vi "E4981_command - 複製.vi"(8 "error in (no error)":errorcluster, 10 "input":T1={"Frequency (1:1kHz)"=1, "Frequency Shift (2: 0%)"=2, "Range"=enum."1p"} {"Frequency Shift (2: 0%)" items=["-2%", "-1%", "0%", "1%", "2%"]; "Frequency (1:1kHz)" items=["120 Hz Frequency", "1 kHz Frequency", "1 MHz Frequency"]}, 11 "command":T3(ring)) -> (0 "error out":errorcluster, 1 "bin":i32, 3 "output":T2={"connectd"=TRUE, "CAP cab"=0.0, "DF  Cab"=0.0} {"CAP cab" format="%#_6p"})   [LabVIEW 2016]
uses:
  meter global.vi
  AOIFramwork/AOIFramework.lvlib
panel:
  in  "reset":bool
  # "CAP DF 電錶作業中"
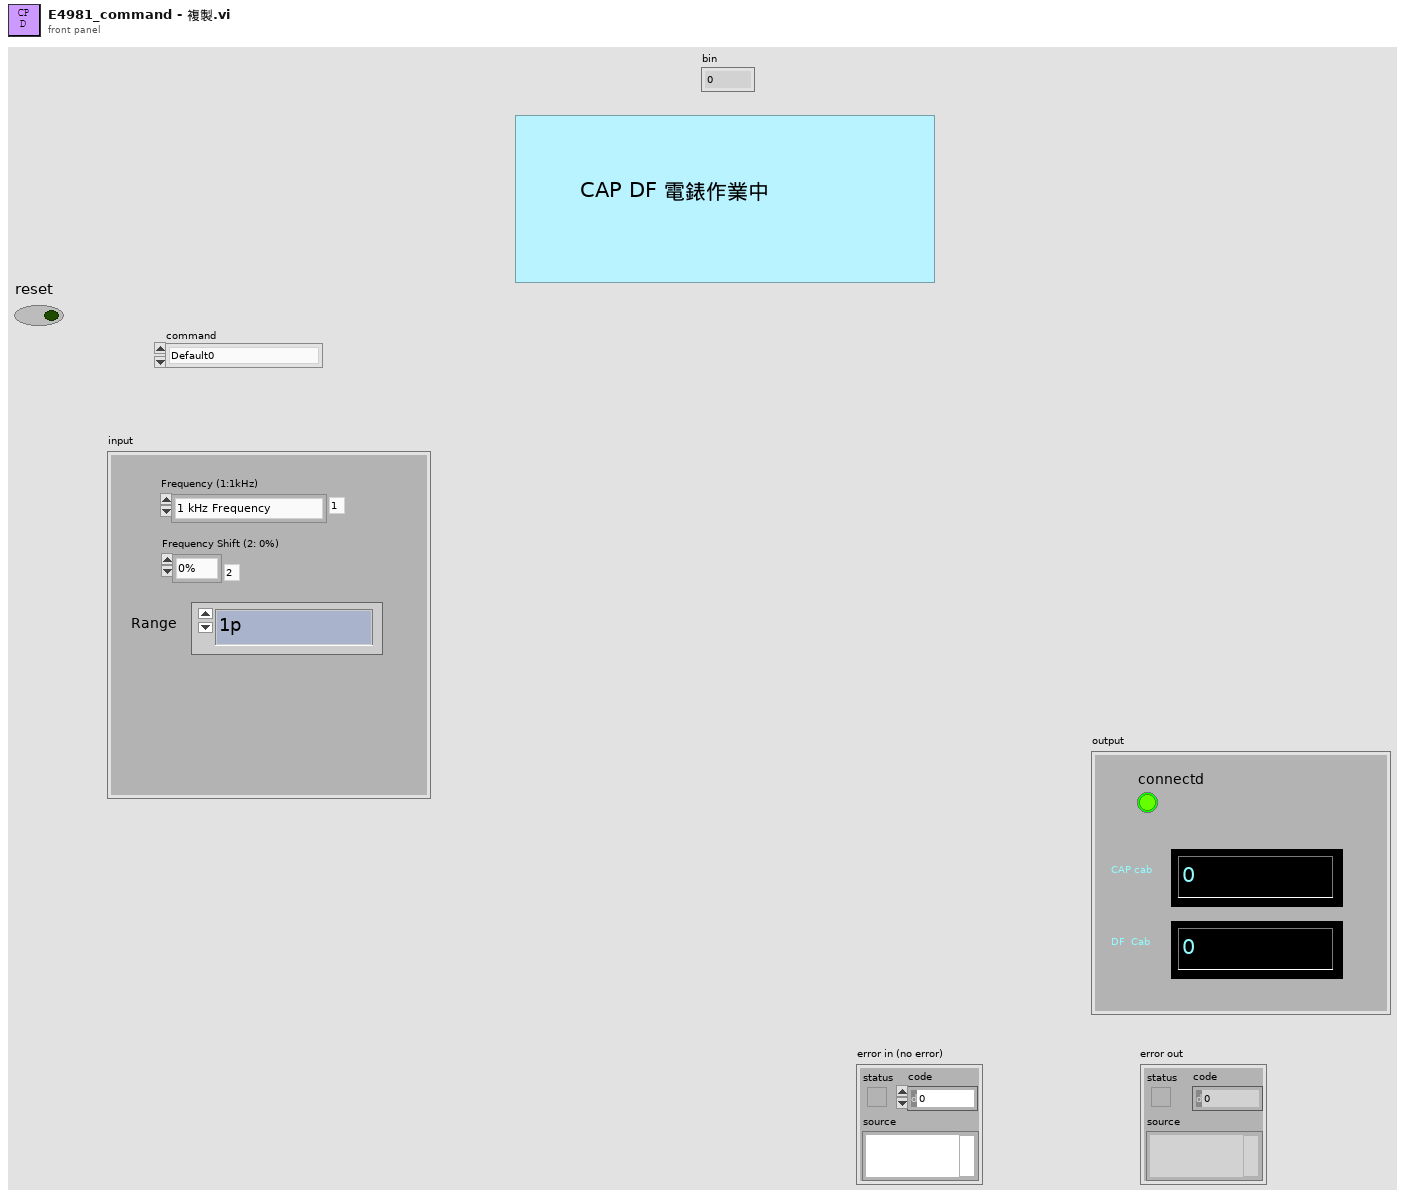
[diagram p1: front panel]
types:
  T1 = cluster{"Frequency (1:1kHz)":u16, "Frequency Shift (2: 0%)":u16, "Range":enum16{"1p", "2.2p", "4.7p", "10p", "22p", "47p", "100p", "220p", "470p", "1n", "2.2n", "4.7n", "10n", "22n", "47n", "100n", "220n", "470n", "1u", "2.2u", "4.7u", "10u", "22u", "47u", "100u", "220u", "470u", "1m", "AUTO", ""}}
  T2 = cluster{"connectd":bool, "CAP cab":dbl, "DF  Cab":dbl}
  T3 = enum16{"Default0", "checkconnect", "int", "changeFEQ", "changeRange", "trigger", "triggerauto"}
  T4 = enum16{"1p", "2.2p", "4.7p", "10p", "22p", "47p", "100p", "220p", "470p", "1n", "2.2n", "4.7n", "10n", "22n", "47n", "100n", "220n", "470n", "1u", "2.2u", "4.7u", "10u", "22u", "47u", "100u", "220u", "470u", "1m", "AUTO", ""}
  T5 = typedef "TypeDef_PNData.ctl" = cluster{"External Diameter":dbl, "Height":dbl, "Range":enum16{"1p", "2.2p", "4.7p", "10p", "22p", "47p", "100p", "220p", "470p", "1n", "2.2n", "4.7n", "10n", "22n", "47n", "100n", "220n", "470n", "1u", "2.2u", "4.7u", "10u", "22u", "47u", "100u", "220u", "470u", "1m", "AUTO", ""}, "DFmin":dbl, "Cap_num":dbl, "F":u16, "BIN3+":dbl, "BIN3- ":dbl, "BIN2+":dbl, "BIN2-":dbl, "BIN1+":dbl, "BIN1-":dbl, "Frequencies":enum16{"120HZ", "1K  HZ", "1M HZ"}, "DFmax":dbl, "Part_5":dbl, "Part_6":dbl, "Part_4":dbl, "Part_8":dbl, "Part_7":dbl, "Par_2":dbl, "part_1":enum16{"DC", "AC"}, "Part_9":dbl, "Part_18":dbl, "Part_15":dbl, "Part_13":dbl, "Part_14":dbl, "Part_16":dbl, "Internal Diameter":dbl}
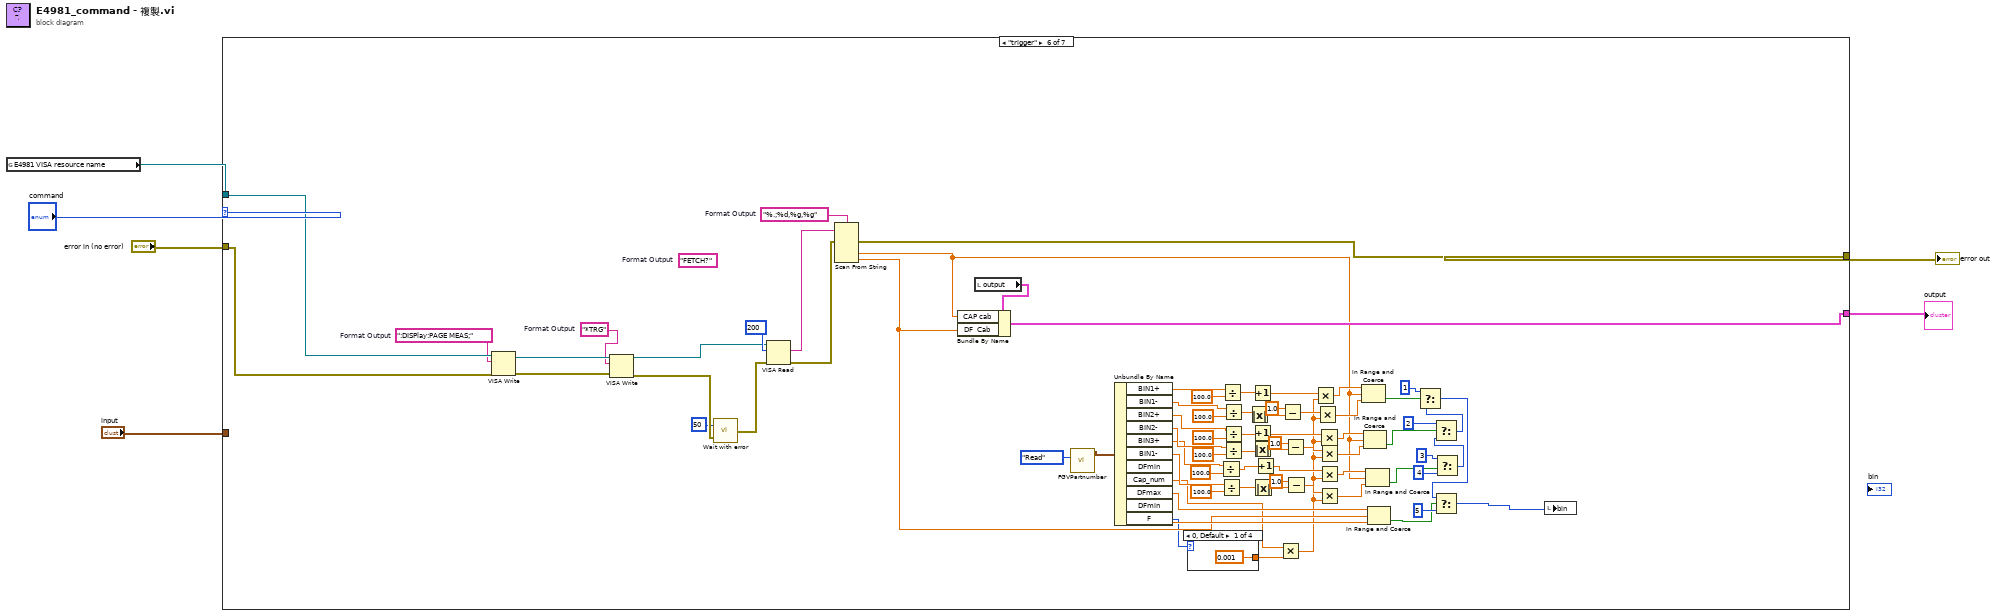
[diagram p0: block diagram]
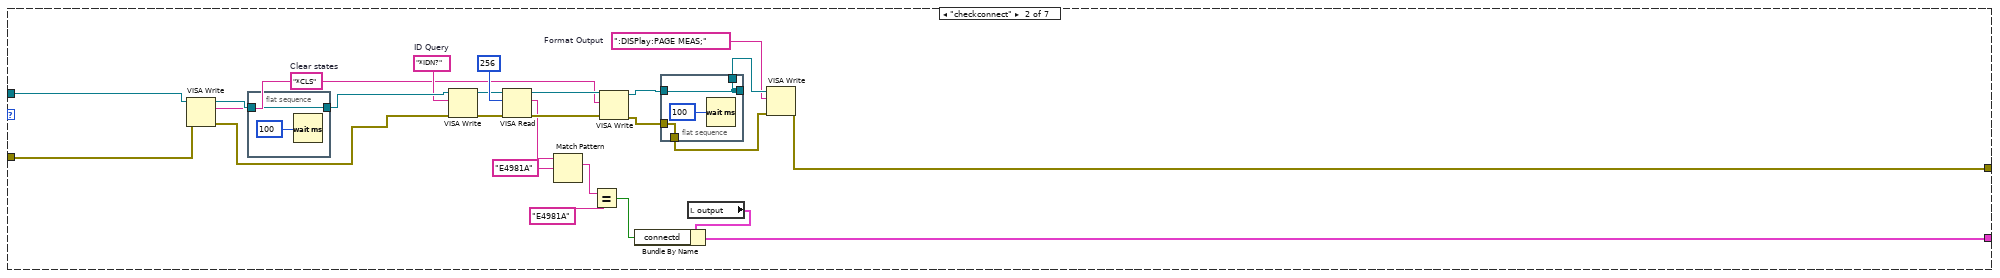
[diagram p3: hidden frame]
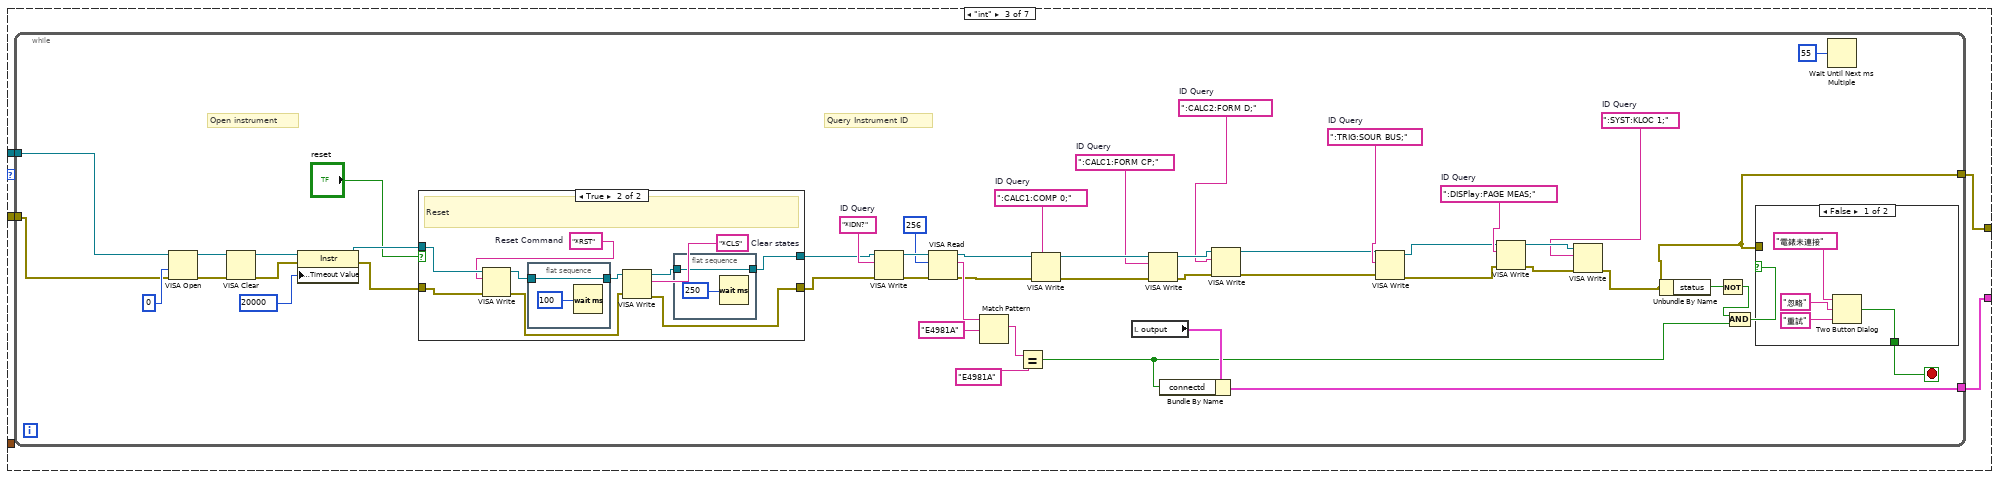
[diagram p4: hidden frame]
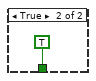
[diagram p6: hidden frame]
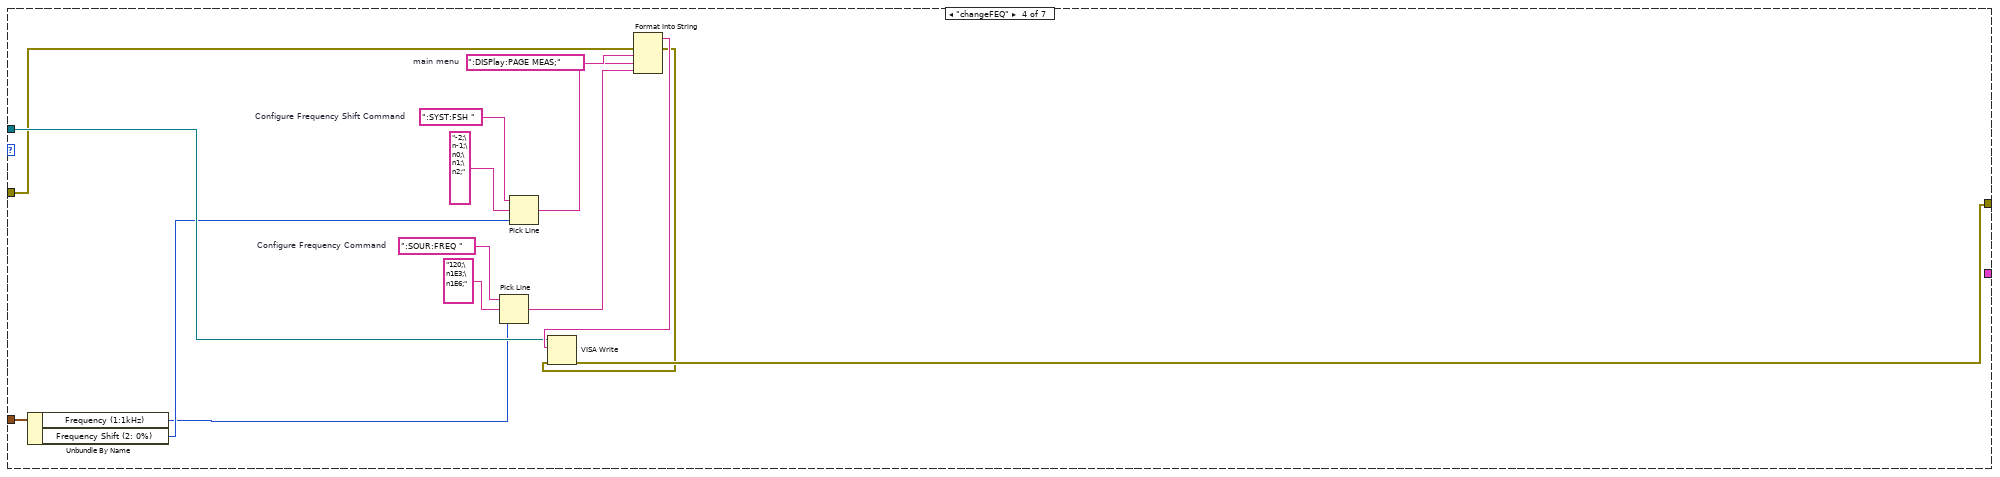
[diagram p7: hidden frame]
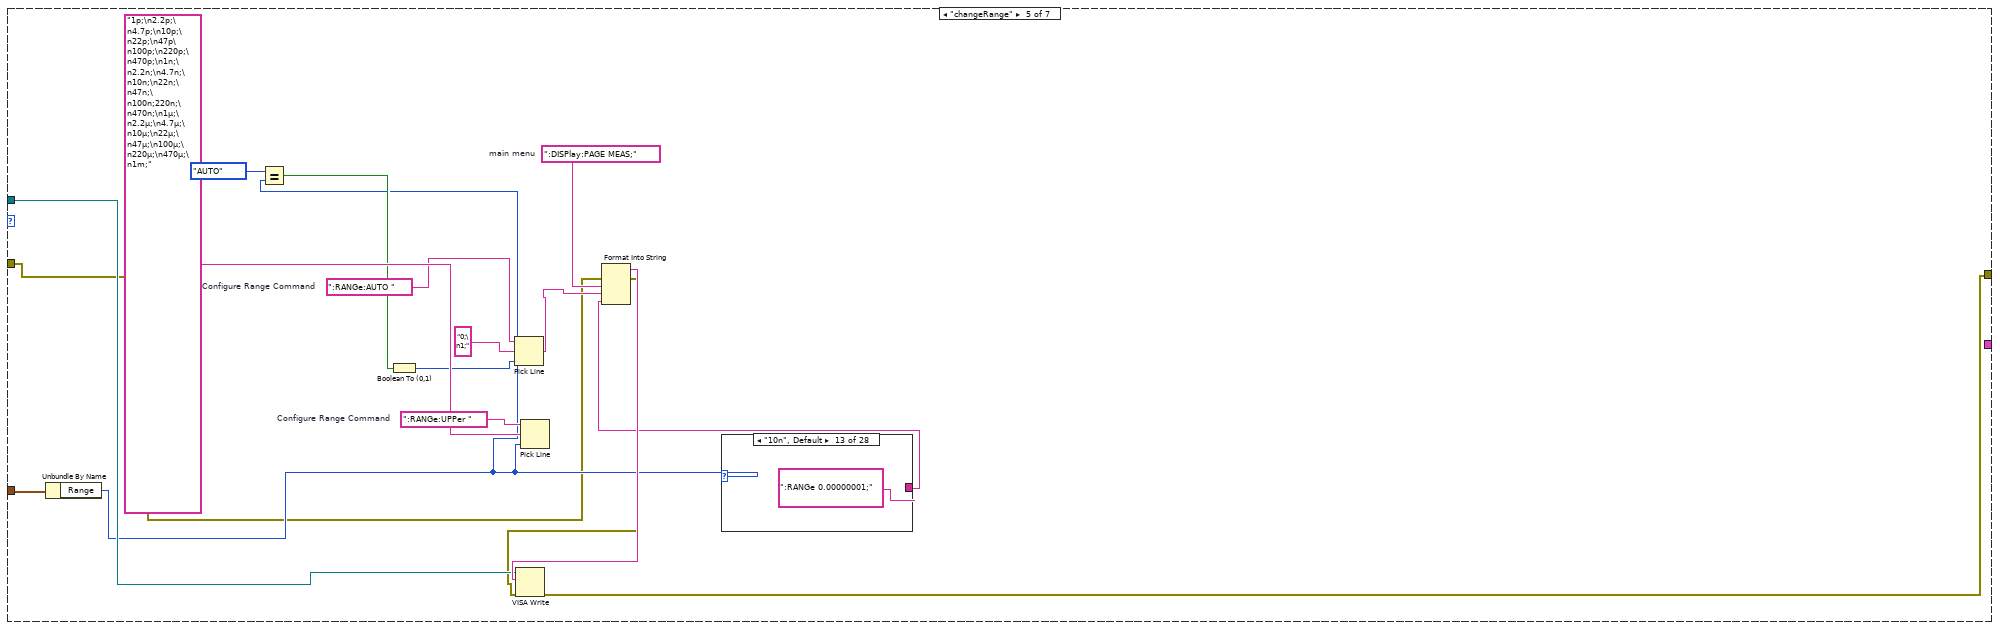
[diagram p8: hidden frame]
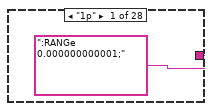
[diagram p9: hidden frame]
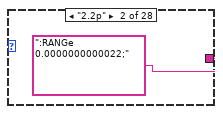
[diagram p10: hidden frame]
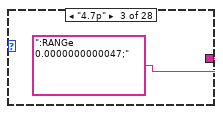
[diagram p11: hidden frame]
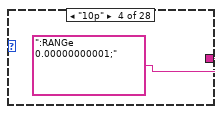
[diagram p12: hidden frame]
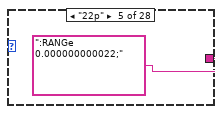
[diagram p13: hidden frame]
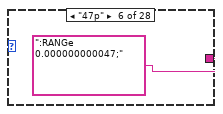
[diagram p14: hidden frame]
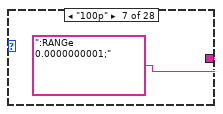
[diagram p15: hidden frame]
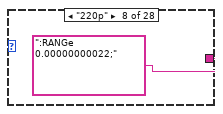
[diagram p16: hidden frame]
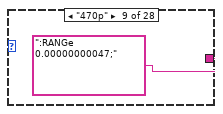
[diagram p17: hidden frame]
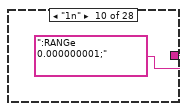
[diagram p18: hidden frame]
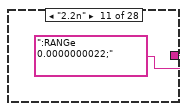
[diagram p19: hidden frame]
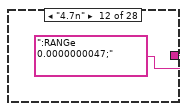
[diagram p20: hidden frame]
diagram:
  n1 = global read "meter global.vi" "E4981 VISA resource name"() -> (w4:refnum<visa-resource-name>)
  n2 = case shown="\"trigger\"" "command" {
    tunnel: "error in (no error)" -> [_ w13 w38 w111 w126 w237 w316]
    tunnel: [_ w12 w40 w115 w129 w232 w258] -> w5
    tunnel: w4 -> [_ w10 w39 w116 w130 w238 w317]
    tunnel: [_ w7 w37 _ _ w235 w314] -> w2
    tunnel: "input" -> [_ _ _ w114 w128 _ _]
    frame "Default0", Default {
    }
    frame "checkconnect" {
      w27 = ":DISPlay:PAGE MEAS;"  # Format Output
      w11 = "*CLS"  # Clear states
      w19 = "*IDN?"  # ID Query
      n3 = VISA Write(VISA resource name=w10, write buffer=w11, error in (no error)=w13) -> (VISA resource name out=w24:refnum<visa-resource-name>, error out=w23:errorcluster)  [unwired: 1 out]
      n4 = flat-sequence {
        tunnel: [w35] -> w22
        tunnel: w24 -> [w35]
        frame #0 {
          n5 = Wait (ms)(milliseconds to wait=u32 100) -> ()  [unwired: 1 out]
        }
      }
      n6 = VISA Write(VISA resource name=w22, write buffer=w19, error in (no error)=w23) -> (VISA resource name out=w15:refnum<visa-resource-name>, error out=w16:errorcluster)  [unwired: 1 out]
      n7 = VISA Read(VISA resource name=w15, byte count=u32 256, error in (no error)=w16) -> (VISA resource name out=w25:refnum<visa-resource-name>, read buffer=w14:string, error out=w26:errorcluster)  [unwired: 1 out]
      n8 = Match Pattern(string=w14, regular expression="E4981A") -> (match substring=w20:string)  [unwired: 1 in, 3 out]
      n9 = Equal?(x=w20, y="E4981A") -> (x = y?=w8:bool)
      n10 = VISA Write(VISA resource name=w25, write buffer=w11, error in (no error)=w26) -> (VISA resource name out=w28:refnum<visa-resource-name>, error out=w29:errorcluster)  [unwired: 1 out]
      n11 = flat-sequence {
        tunnel: [w32] -> _
        tunnel: w28 -> [w32]
        tunnel: w29 -> [w33]
        tunnel: [w33] -> w30
        tunnel: [w32] -> w31
        frame #0 {
          n12 = Wait (ms)(milliseconds to wait=u32 100) -> ()  [unwired: 1 out]
        }
      }
      n13 = local read "output"() -> (w9:T2)
      n14 = Bundle By Name(cluster=w9, "connectd"=w8) -> (w7:T2)
      n15 = VISA Write(VISA resource name=w31, write buffer=w27, error in (no error)=w30) -> (error out=w12:errorcluster)  [unwired: 2 out]
    }
    frame "int" {
      n16 = while {
        tunnel: [w46] -> w40
        tunnel: w39 -> [w45]
        tunnel: w38 -> [w44]
        tunnel: [w41] -> w37
        stop <- w73 stop-if-true
        w54 = ":TRIG:SOUR BUS;"  # ID Query
        w57 = ":SYST:KLOC 1;"  # ID Query
        w60 = ":DISPlay:PAGE MEAS;"  # ID Query
        w61 = ":CALC2:FORM D;"  # ID Query
        w62 = ":CALC1:FORM CP;"  # ID Query
        w71 = ":CALC1:COMP 0;"  # ID Query
        w77 = "*IDN?"  # ID Query
        # "Query Instrument ID"
        # "Open instrument"
        n17 = VISA Open(access mode=u32 0, error in (no error)=w44, VISA resource name=w45) -> (VISA resource name=w86:refnum<visa-resource-name>, error out=w85:errorcluster)  [unwired: 2 in]
        n18 = VISA Clear(VISA resource name=w86, error in (no error)=w85) -> (VISA resource name out=w84:refnum<visa-resource-name>, error out=w83:errorcluster)
        n19 = property class="Instr"(reference=w84, error in=w83, "General Settings:Timeout Value"=u32 20000) -> (reference out=w50:refnum<visa-resource-name>, error out=w48:errorcluster)
        n20 = case shown="True" "reset" {
          tunnel: [w90 w95] -> w51
          tunnel: w50 -> [w90 w100]
          tunnel: [w89 w93] -> w49
          tunnel: w48 -> [w89 w92]
          frame False {
          }
          frame True {
            w91 = "*CLS"  # Clear states
            w99 = "*RST"  # Reset Command
            # "Reset"
            n21 = VISA Write(VISA resource name=w100, write buffer=w99, error in (no error)=w92) -> (VISA resource name out=w97:refnum<visa-resource-name>, error out=w94:errorcluster)  [unwired: 1 out]
            n22 = flat-sequence {
              tunnel: [w103] -> w98
              tunnel: w97 -> [w103]
              frame #0 {
                n23 = Wait (ms)(milliseconds to wait=u32 100) -> ()  [unwired: 1 out]
              }
            }
            n24 = VISA Write(VISA resource name=w98, write buffer=w91, error in (no error)=w94) -> (VISA resource name out=w96:refnum<visa-resource-name>, error out=w93:errorcluster)  [unwired: 1 out]
            n25 = flat-sequence {
              tunnel: [w101] -> w95
              tunnel: w96 -> [w101]
              frame #0 {
                n26 = Wait (ms)(milliseconds to wait=u32 250) -> ()  [unwired: 1 out]
              }
            }
          }
        }
        n27 = VISA Write(VISA resource name=w51, write buffer=w77, error in (no error)=w49) -> (VISA resource name out=w81:refnum<visa-resource-name>, error out=w80:errorcluster)  [unwired: 1 out]
        n28 = VISA Read(VISA resource name=w81, byte count=u32 256, error in (no error)=w80) -> (VISA resource name out=w69:refnum<visa-resource-name>, read buffer=w82:string, error out=w70:errorcluster)  [unwired: 1 out]
        n29 = Match Pattern(string=w82, regular expression="E4981A") -> (match substring=w75:string)  [unwired: 1 in, 3 out]
        n30 = Equal?(x=w75, y="E4981A") -> (x = y?=w42:bool)
        n31 = VISA Write(VISA resource name=w69, write buffer=w71, error in (no error)=w70) -> (VISA resource name out=w66:refnum<visa-resource-name>, error out=w65:errorcluster)  [unwired: 1 out]
        n32 = local read "output"() -> (w43:T2)
        n33 = VISA Write(VISA resource name=w66, write buffer=w62, error in (no error)=w65) -> (VISA resource name out=w63:refnum<visa-resource-name>, error out=w64:errorcluster)  [unwired: 1 out]
        n34 = Bundle By Name(cluster=w43, "connectd"=w42) -> (w41:T2)
        n35 = VISA Write(VISA resource name=w63, write buffer=w61, error in (no error)=w64) -> (VISA resource name out=w53:refnum<visa-resource-name>, error out=w52:errorcluster)  [unwired: 1 out]
        n36 = VISA Write(VISA resource name=w53, write buffer=w54, error in (no error)=w52) -> (VISA resource name out=w56:refnum<visa-resource-name>, error out=w55:errorcluster)  [unwired: 1 out]
        n37 = VISA Write(VISA resource name=w56, write buffer=w60, error in (no error)=w55) -> (VISA resource name out=w58:refnum<visa-resource-name>, error out=w59:errorcluster)  [unwired: 1 out]
        n38 = VISA Write(VISA resource name=w58, write buffer=w57, error in (no error)=w59) -> (error out=w46:errorcluster)  [unwired: 2 out]
        n39 = Unbundle By Name(w46) -> ("status"=w68:bool)
        n40 = Not(x=w68) -> (.not. x?=w67:bool)
        n41 = And(x=w67, y=w42) -> (x .and. y?=w76:bool)
        n42 = case shown="False" w76 {
          tunnel: [w107 TRUE ("cancel 2")] -> w73
          tunnel: w46 -> [_ _]
          frame False {
            n43 = Two Button Dialog(message="電錶未連接", 1:"重試" ("T button name (\"OK\")"), 2:"忽略" ("F button name (\"Cancel\")")) -> (T button?=w107:bool)
          }
          frame True {
          }
        }
        n44 = Wait Until Next ms Multiple(millisecond multiple=u32 55) -> ()  [unwired: 1 out]
      }
    }
    frame "changeFEQ" {
      w120 = ":DISPlay:PAGE MEAS;"  # main menu
      w121 = ":SYST:FSH "  # Configure Frequency Shift Command
      w122 = ":SOUR:FREQ "  # Configure Frequency Command
      n45 = Unbundle By Name(w114) -> ("Frequency (1:1kHz)"=w112:u16, "Frequency Shift (2: 0%)"=w113:u16)
      n46 = Pick Line(string ("")=w122, multi-line string="120;\n1E3;\n1E6;", line index=w112) -> (output string=w118:string)
      n47 = Pick Line(string ("")=w121, multi-line string="-2;\n-1;\n0;\n1;\n2;", line index=w113) -> (output string=w119:string)
      n48 = Format Into String(error in=w111, w120, w119, w118) -> (resulting string=w117:string, error out=w110:errorcluster)  [unwired: 2 in]
      n49 = VISA Write(VISA resource name=w116, write buffer=w117, error in (no error)=w110) -> (error out=w115:errorcluster)  [unwired: 2 out]
    }
    frame "changeRange" {
      w139 = ":RANGe:UPPer "  # Configure Range Command
      w136 = ":RANGe:AUTO "  # Configure Range Command
      w141 = ":DISPlay:PAGE MEAS;"  # main menu
      n50 = Unbundle By Name(w128) -> ("Range"=w127:T4)
      n51 = Equal?(x=T4."AUTO", y=w127) -> (x = y?=w134:bool)
      n52 = Boolean To (0,1)(Boolean=w134) -> (0, 1=w133:i16)
      n53 = Pick Line(string ("")=w136, multi-line string="0;\n1;", line index=w133) -> (output string=w132:string)
      n54 = Pick Line(string ("")=w139, multi-line string="1p;\n2.2p;\n4.7p;\n10p;\n22p;\n47p\n100p;\n220p;\n470p;\n1n;\n2.2n;\n4.7n;\n10n;\n22n;\n47n;\n100n;220n;\n470n;\n1μ;\n2.2μ;\n4.7μ;\n10μ;\n22μ;\n47μ;\n100μ;\n220μ;\n470μ;\n1m;", line index=w127) -> ()  [unwired: 1 out]
      n55 = case shown="\"10n\", Default" w127 {
        tunnel: [":RANGe 0.000000000001;" ("Configure Range Command") ":RANGe 0.0000000000022;" ("Configure Range Command") ":RANGe 0.0000000000047;" ("Configure Range Command") ":RANGe 0.00000000001;" ("Configure Range Command") ":RANGe 0.000000000022;" ("Configure Range Command") ":RANGe 0.000000000047;" ("Configure Range Command") ":RANGe 0.0000000001;" ("Configure Range Command") ":RANGe 0.00000000022;" ("Configure Range Command") ":RANGe 0.00000000047;" ("Configure Range Command") ":RANGe 0.000000001;" ("Configure Range Command") ":RANGe 0.0000000022;" ("Configure Range Command") ":RANGe 0.0000000047;" ("Configure Range Command") ":RANGe 0.00000001;" ("Configure Range Command") ":RANGe 0.000000022;" ("Configure Range Command") ":RANGe 0.000000047;" ("Configure Range Command") ":RANGe 0.0000001;" ("Configure Range Command") ":RANGe 0.00000022;" ("Configure Range Command") ":RANGe 0.00000047;" ("Configure Range Command") ":RANGe 0.000001;" ("Configure Range Command") ":RANGe 0.0000022;" ("Configure Range Command") ":RANGe 0.0000047;" ("Configure Range Command") ":RANGe 0.00001;" ("Configure Range Command") ":RANGe 0.000022;" ("Configure Range Command") ":RANGe 0.000047;" ("Configure Range Command") ":RANGe 0.0001;" ("Configure Range Command") ":RANGe 0.00022;" ("Configure Range Command") ":RANGe 0.00047;" ("Configure Range Command") ":RANGe 0.001;" ("Configure Range Command")] -> w131
        frame "1p" {
        }
        frame "2.2p" {
        }
        frame "4.7p" {
        }
        frame "10p" {
        }
        frame "22p" {
        }
        frame "47p" {
        }
        frame "100p" {
        }
        frame "220p" {
        }
        frame "470p" {
        }
        frame "1n" {
        }
        frame "2.2n" {
        }
        frame "4.7n" {
        }
        frame "10n", Default {
        }
        frame "22n" {
        }
        frame "47n" {
        }
        frame "100n" {
        }
        frame "220n" {
        }
        frame "470n" {
        }
        frame "1u" {
        }
        frame "2.2u" {
        }
        frame "4.7u" {
        }
        frame "10u" {
        }
        frame "22u" {
        }
        frame "47u" {
        }
        frame "100u" {
        }
        frame "220u" {
        }
        frame "470u" {
        }
        frame "1m" {
        }
      }
      n56 = Format Into String(error in=w126, w141, w132, w131) -> (resulting string=w140:string, error out=w125:errorcluster)  [unwired: 2 in]
      n57 = VISA Write(VISA resource name=w130, write buffer=w140, error in (no error)=w125) -> (error out=w129:errorcluster)  [unwired: 2 out]
    }
    frame "trigger" {
      w234 = ":DISPlay:PAGE MEAS;"  # Format Output
      (unwired) "FETCH?"  # Format Output
      w239 = "*TRG"  # Format Output
      w243 = "%.;%d,%g,%g"  # Format Output
      n58 = VISA Write(VISA resource name=w238, write buffer=w234, error in (no error)=w237) -> (VISA resource name out=w240:refnum<visa-resource-name>, error out=w241:errorcluster)  [unwired: 1 out]
      n59 = VISA Write(VISA resource name=w240, write buffer=w239, error in (no error)=w241) -> (VISA resource name out=w242:refnum<visa-resource-name>, error out=w172:errorcluster)  [unwired: 1 out]
      n60 = call "Wait with error.vi"("error in (no error)"=w172, "milliseconds to wait"=u32 50) -> ("error out"=w171:errorcluster)
      n61 = VISA Read(VISA resource name=w242, byte count=u32 200, error in (no error)=w171) -> (read buffer=w244:string, error out=w233:errorcluster)  [unwired: 2 out]
      n62 = Scan From String(format string=w243, input string=w244, error in=w233) -> (error out=w232:errorcluster, output 2=w178:dbl, output 3=w177:dbl)  [unwired: 5 in, 2 out]
      n63 = local read "output"() -> (w236:T2)
      n64 = Bundle By Name(cluster=w236, "CAP cab"=w178, "DF  Cab"=w177) -> (w235:T2)
      n65 = call "FGVPartnumber.vi"("Enum"=enum16{"Write", "Read"}."Read") -> ("UnitParamiterCluster out"=w230:T5)  [unwired: 10 in]
      n66 = Unbundle By Name(w230) -> ("BIN1+"=w229:dbl, "BIN1-"=w226:dbl, "BIN2+"=w224:dbl, "BIN2-"=w222:dbl, "BIN3+"=w220:dbl, "BIN1-"=w218:dbl, "Cap_num"=w174:dbl, "DFmax"=w193:dbl, "DFmin"=w192:dbl, "F"=w176:u16)  [unwired: 1 out]
      n67 = case shown="0, Default" w176 {
        tunnel: [0.001 1e-06 1e-09 1e-12] -> w175
        frame 0, Default {
        }
        frame 1 {
        }
        frame 2 {
        }
        frame 3 {
        }
      }
      n68 = Divide(x=w220, y=100.0) -> (x/y=w206:dbl)
      n69 = Divide(x=w218, y=100.0) -> (x/y=w208:dbl)
      n70 = Divide(x=w229, y=100.0) -> (x/y=w217:dbl)
      n71 = Divide(x=w226, y=100.0) -> (x/y=w216:dbl)
      n72 = Divide(x=w224, y=100.0) -> (x/y=w207:dbl)
      n73 = Divide(x=w222, y=100.0) -> (x/y=w211:dbl)
      n74 = Absolute Value(x=w216) -> (abs(x)=w215:dbl)
      n75 = Increment(x=w217) -> (x+1=w205:dbl)
      n76 = Increment(x=w207) -> (x+1=w203:dbl)
      n77 = Absolute Value(x=w211) -> (abs(x)=w212:dbl)
      n78 = Absolute Value(x=w208) -> (abs(x)=w210:dbl)
      n79 = Increment(x=w206) -> (x+1=w201:dbl)
      n80 = Multiply(x=w174, y=w175) -> (x*y=w173:dbl)
      n81 = Subtract(x=1.0, y=w215) -> (x-y=w204:dbl)
      n82 = Subtract(x=1.0, y=w212) -> (x-y=w202:dbl)
      n83 = Subtract(x=1.0, y=w210) -> (x-y=w200:dbl)
      n84 = Multiply(x=w205, y=w173) -> (x*y=w199:dbl)
      n85 = Multiply(x=w204, y=w173) -> (x*y=w198:dbl)
      n86 = Multiply(x=w203, y=w173) -> (x*y=w197:dbl)
      n87 = Multiply(x=w202, y=w173) -> (x*y=w196:dbl)
      n88 = Multiply(x=w201, y=w173) -> (x*y=w195:dbl)
      n89 = Multiply(x=w200, y=w173) -> (x*y=w194:dbl)
      n90 = In Range and Coerce(upper limit=w199, x=w178, lower limit=w198) -> (In Range?=w191:bool)  [unwired: 1 out]
      n91 = In Range and Coerce(upper limit=w197, x=w178, lower limit=w196) -> (In Range?=w183:bool)  [unwired: 1 out]
      n92 = In Range and Coerce(upper limit=w195, x=w178, lower limit=w194) -> (In Range?=w185:bool)  [unwired: 1 out]
      n93 = In Range and Coerce(upper limit=w193, x=w177, lower limit=w192) -> (In Range?=w186:bool)  [unwired: 1 out]
      n94 = Select(t=3, s=w185, f=4) -> (s? t:f=w184:i32)
      n95 = Select(t=2, s=w183, f=w184) -> (s? t:f=w182:i32)
      n96 = Select(t=1, s=w191, f=w182) -> (s? t:f=w180:i32)
      n97 = Select(t=w180, s=w186, f=5) -> (s? t:f=w179:i32)
      n98 = local write "bin"(w179) -> ()
    }
    frame "triggerauto" {
      w313 = enum16{"Write", "Read"}."Read"  # Enum
      (unwired) "FETCH?"  # Format Output
      w318 = "*TRG"  # Format Output
      w322 = "%.;%d,%g,%g"  # Format Output
      n99 = disable-structure shown="Disabled" {
        disable-tunnel: [w333 w334] -> w320
        disable-tunnel: [w332 w335] -> w319
        disable-tunnel: w317 -> [w331 w335]
        disable-tunnel: w316 -> [w330 w334]
        frame Disabled {
          w329 = ":DISPlay:PAGE MEAS;"  # Format Output
          n100 = VISA Write(VISA resource name=w331, write buffer=w329, error in (no error)=w330) -> (VISA resource name out=w332:refnum<visa-resource-name>, error out=w333:errorcluster)  [unwired: 1 out]
        }
        frame Enabled {
        }
      }
      n101 = VISA Write(VISA resource name=w319, write buffer=w318, error in (no error)=w320) -> (VISA resource name out=w321:refnum<visa-resource-name>, error out=w252:errorcluster)  [unwired: 1 out]
      n102 = call "Wait with error.vi"("error in (no error)"=w252, "milliseconds to wait"=u32 50) -> ("error out"=w251:errorcluster)
      n103 = VISA Read(VISA resource name=w321, byte count=u32 200, error in (no error)=w251) -> (read buffer=w323:string, error out=w259:errorcluster)  [unwired: 2 out]
      n104 = Scan From String(format string=w322, input string=w323, error in=w259) -> (error out=w258:errorcluster, output 2=w263:dbl, output 3=w262:dbl)  [unwired: 5 in, 2 out]
      n105 = local read "output"() -> (w315:T2)
      n106 = Bundle By Name(cluster=w315, "CAP cab"=w263, "DF  Cab"=w262) -> (w314:T2)
      n107 = call "FGVPartnumber.vi"("Enum"=w313) -> ("UnitParamiterCluster out"=w312:T5)  [unwired: 10 in]
      n108 = Unbundle By Name(w312) -> ("BIN1+"=w311:dbl, "BIN1-"=w308:dbl, "BIN2+"=w306:dbl, "BIN2-"=w304:dbl, "BIN3+"=w302:dbl, "BIN1-"=w300:dbl, "Cap_num"=w254:dbl, "DFmax"=w275:dbl, "DFmin"=w274:dbl, "F"=w255:u16)  [unwired: 1 out]
      n109 = Divide(x=w302, y=100.0) -> (x/y=w288:dbl)
      n110 = Divide(x=w300, y=100.0) -> (x/y=w290:dbl)
      n111 = Divide(x=w311, y=100.0) -> (x/y=w299:dbl)
      n112 = Divide(x=w308, y=100.0) -> (x/y=w298:dbl)
      n113 = Divide(x=w306, y=100.0) -> (x/y=w289:dbl)
      n114 = Divide(x=w304, y=100.0) -> (x/y=w293:dbl)
      n115 = case shown="0, Default" w255 {
        tunnel: [0.001 1e-06 1e-09 1e-12] -> w256
        frame 0, Default {
        }
        frame 1 {
        }
        frame 2 {
        }
        frame 3 {
        }
      }
      n116 = Absolute Value(x=w298) -> (abs(x)=w297:dbl)
      n117 = Increment(x=w299) -> (x+1=w287:dbl)
      n118 = Increment(x=w289) -> (x+1=w285:dbl)
      n119 = Absolute Value(x=w293) -> (abs(x)=w294:dbl)
      n120 = Absolute Value(x=w290) -> (abs(x)=w292:dbl)
      n121 = Increment(x=w288) -> (x+1=w283:dbl)
      n122 = Subtract(x=1.0, y=w297) -> (x-y=w286:dbl)
      n123 = Subtract(x=1.0, y=w294) -> (x-y=w284:dbl)
      n124 = Subtract(x=1.0, y=w292) -> (x-y=w282:dbl)
      n125 = Multiply(x=w254, y=w256) -> (x*y=w253:dbl)
      n126 = Multiply(x=w287, y=w253) -> (x*y=w281:dbl)
      n127 = Multiply(x=w286, y=w253) -> (x*y=w280:dbl)
      n128 = Multiply(x=w285, y=w253) -> (x*y=w279:dbl)
      n129 = Multiply(x=w284, y=w253) -> (x*y=w278:dbl)
      n130 = Multiply(x=w283, y=w253) -> (x*y=w277:dbl)
      n131 = Multiply(x=w282, y=w253) -> (x*y=w276:dbl)
      n132 = In Range and Coerce(upper limit=w281, x=w263, lower limit=w280) -> (In Range?=w273:bool)  [unwired: 1 out]
      n133 = In Range and Coerce(upper limit=w279, x=w263, lower limit=w278) -> (In Range?=w265:bool)  [unwired: 1 out]
      n134 = In Range and Coerce(upper limit=w277, x=w263, lower limit=w276) -> (In Range?=w267:bool)  [unwired: 1 out]
      n135 = In Range and Coerce(upper limit=w275, x=w262, lower limit=w274) -> (In Range?=w268:bool)  [unwired: 1 out]
      n136 = Select(t=3, s=w267, f=4) -> (s? t:f=w266:i32)
      n137 = Select(t=2, s=w265, f=w266) -> (s? t:f=w264:i32)
      n138 = Select(t=1, s=w273, f=w264) -> (s? t:f=w260:i32)
      n139 = Select(t=w260, s=w268, f=5) -> (s? t:f=w257:i32)
      n140 = local write "bin"(w257) -> ()
    }
  }
  "error out" <- w5
  "output" <- w2
